vi "graph_draw.vi"(2 "yi":dbl, 3 "element":cluster{"xi":dbl[], "yi":dbl[]}, 4 "map_in":cluster{"xi":dbl[], "yi":dbl[]}, 5 "xy_in":cluster{"xi":dbl[], "yi":dbl[]}, 6 "xi":dbl) -> (0 "XY Graph":cluster{"xi":dbl[], "yi":dbl[]}[](graph), 1 "pos_o":cluster{"xo":dbl[], "yo":dbl[]})   [LabVIEW 2015]
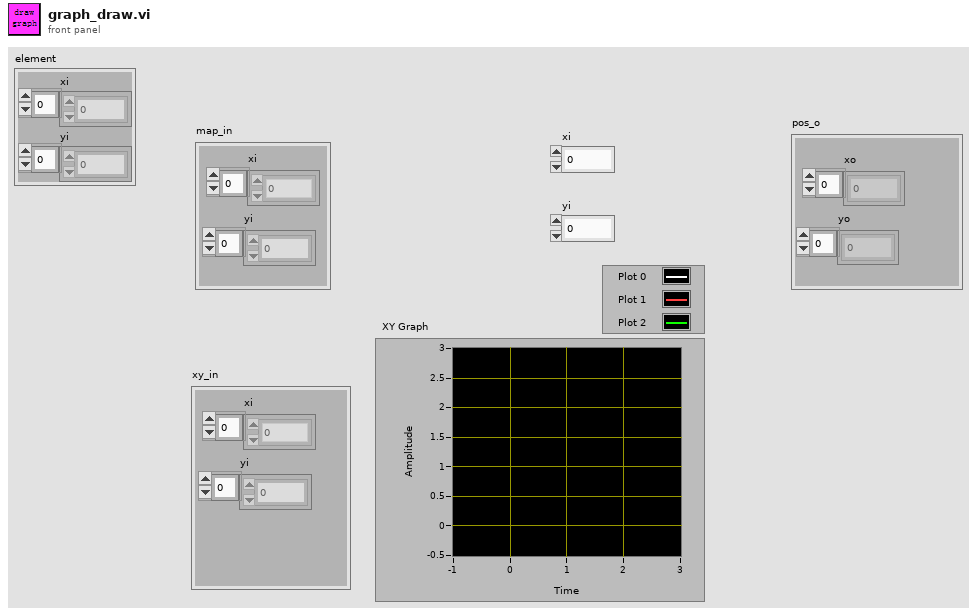
[diagram p1: front panel]
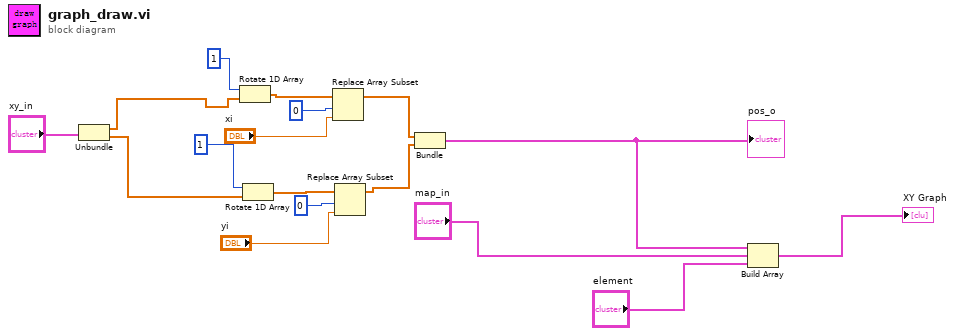
[diagram p0: block diagram]
diagram:
  n1 = Unbundle("xy_in") -> ("xi"=w6:dbl[], "yi"=w5:dbl[])
  n2 = Rotate 1D Array(1:w6, 2:1) -> (0:w15:dbl[])
  n3 = Rotate 1D Array(1:w5, 2:1) -> (0:w14:dbl[])
  n4 = Replace Array Subset(array=w15, new element="xi", index=0) -> (w9:dbl[])
  n5 = Replace Array Subset(array=w14, new element="yi", index=0) -> (w8:dbl[])
  n6 = Bundle(w9, w8) -> (w4:cluster{dbl[], dbl[]})  [unwired: 1 in]
  "pos_o" <- w4
  n7 = Build Array(w4, "map_in", "element") -> (→"XY Graph":cluster{"xi":dbl[], "yi":dbl[]}[])
